vi "oef11.vi"() -> ()   [LabVIEW 2021]
uses:
  <vilib>/httpClient/LabVIEWHTTPClient.lvlib
panel:
  out "before substring":string
  out "match substring":string
  out "after substring":string
  in  "word":string
  out "headers":string
  out "body":string
  in  "String":string
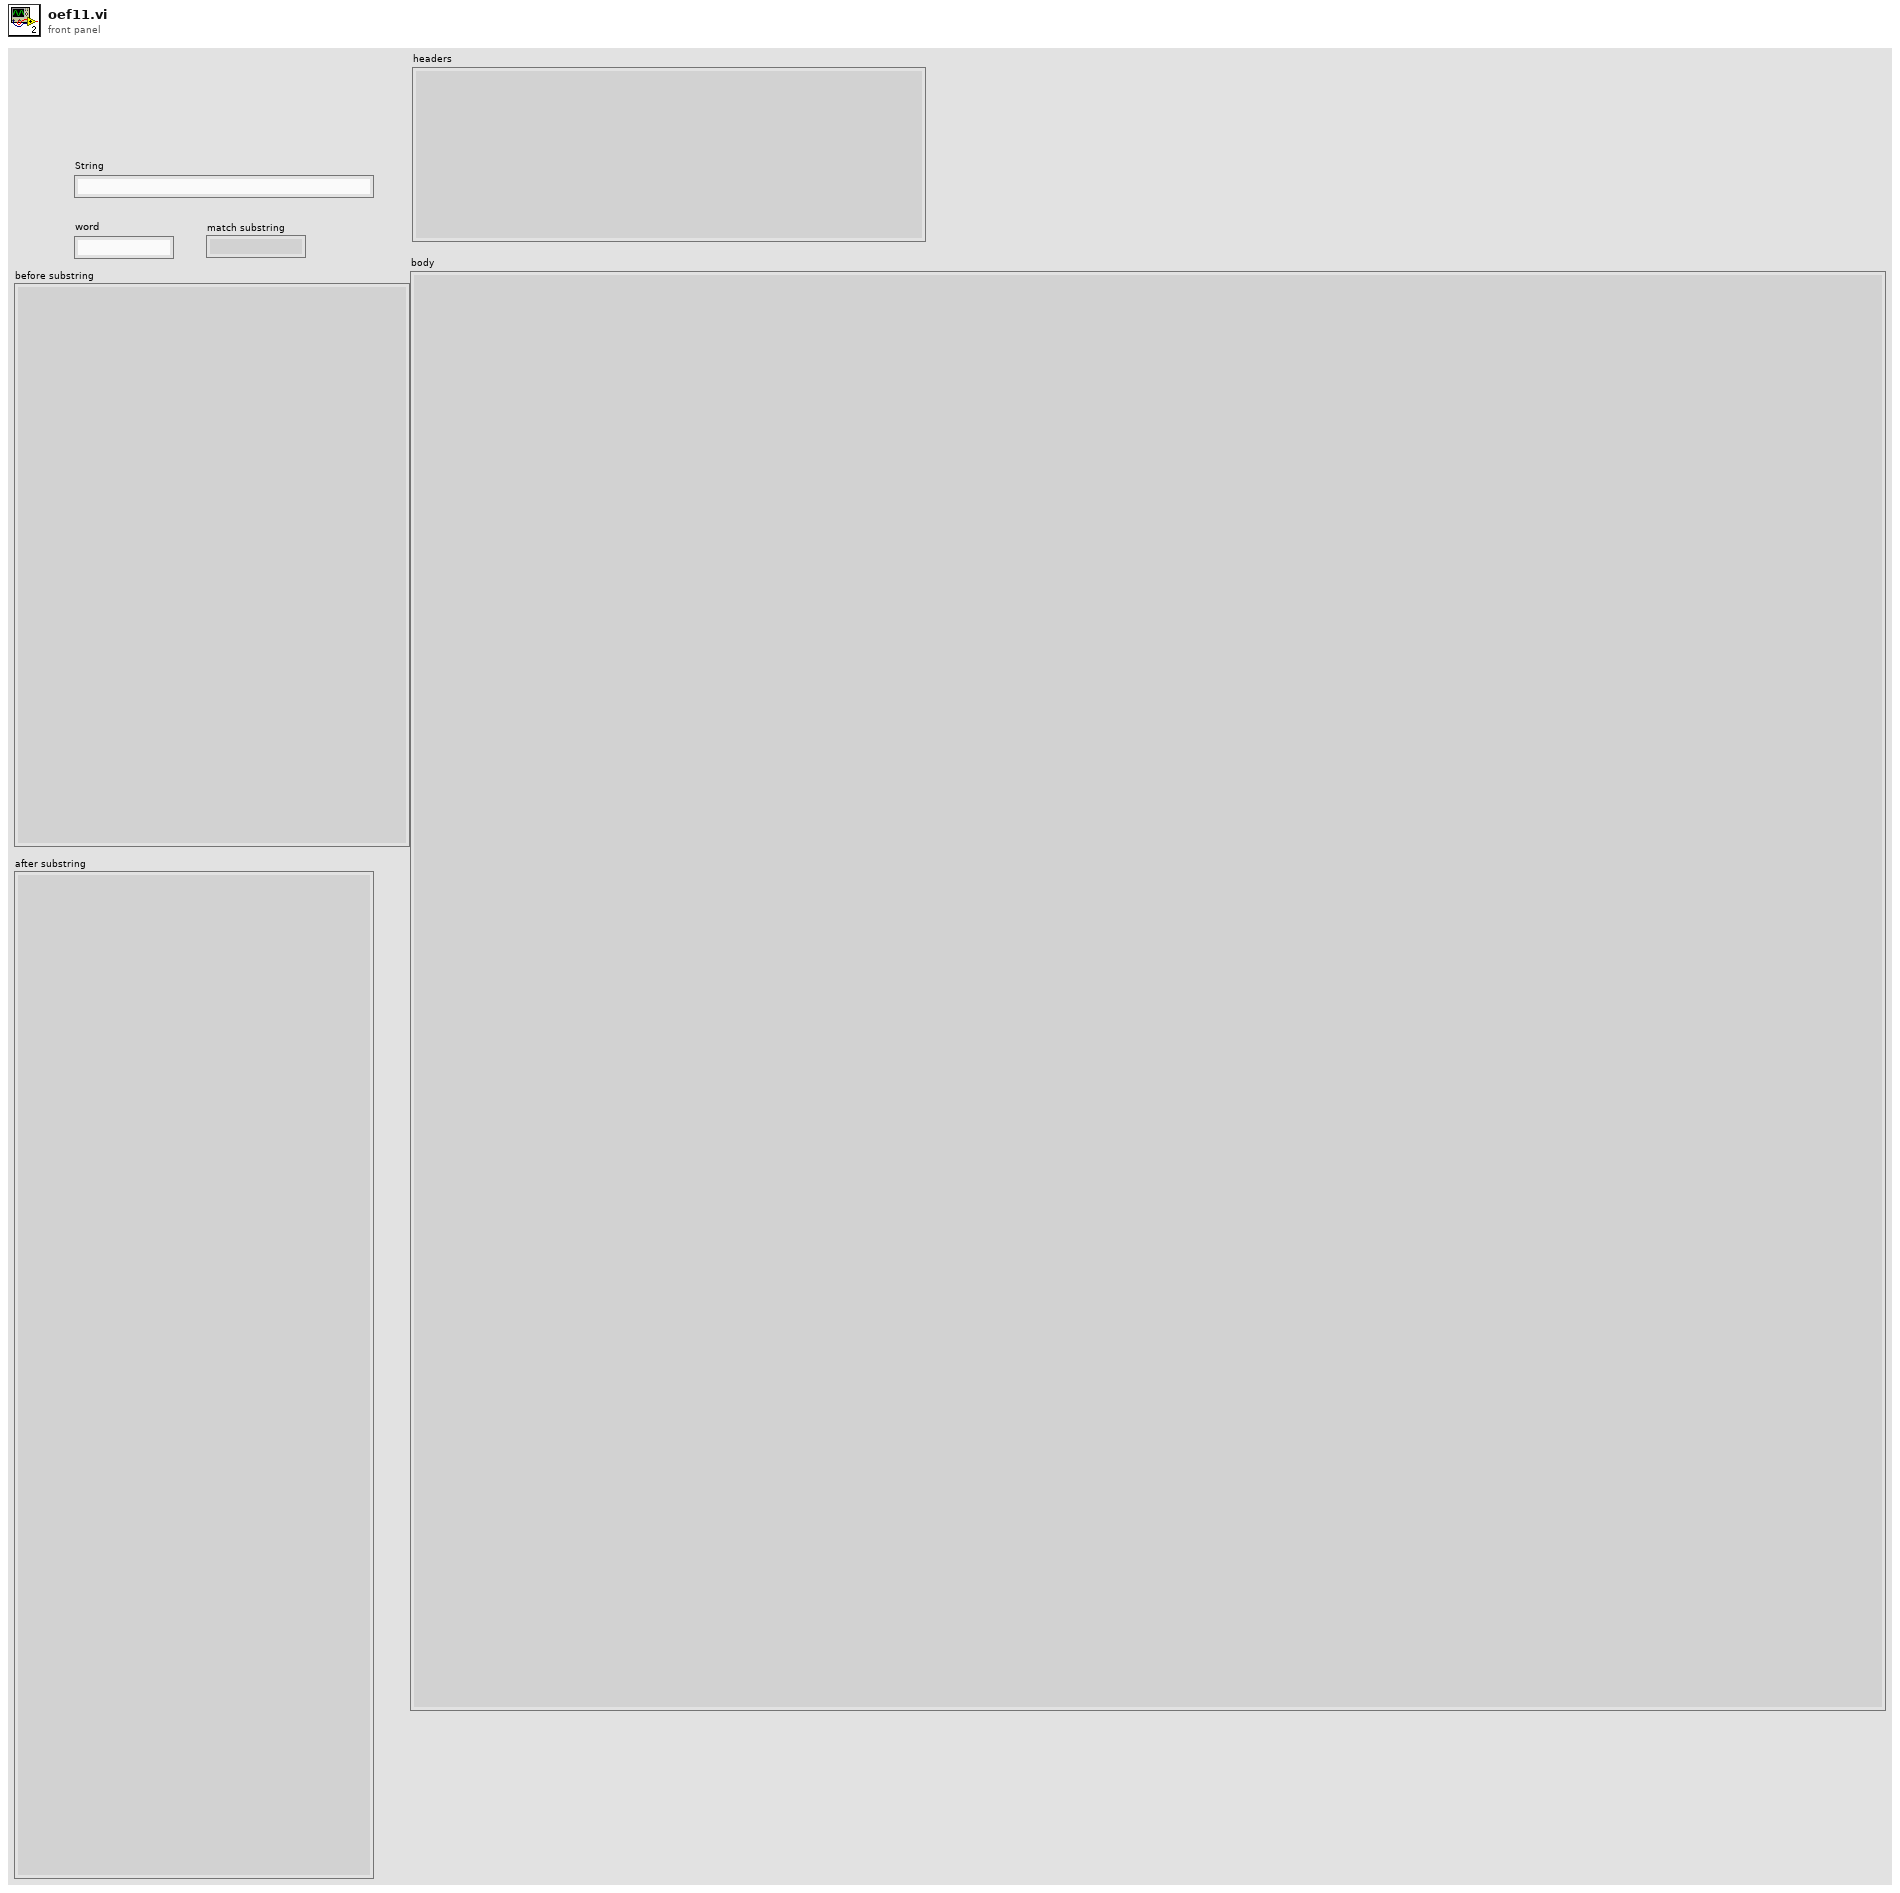
[diagram p1: front panel]
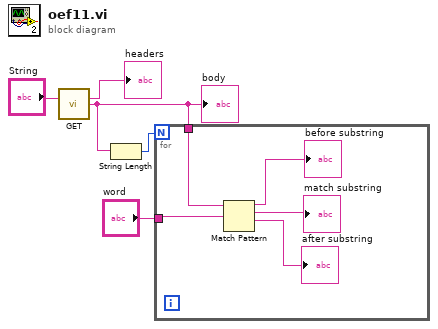
[diagram p0: block diagram]
diagram:
  n1 = call <vilib>:"GET.vi"("url"="String") -> ("headers"=→"headers":string, "body"=w2:string)  [unwired: 11 in, 2 out]
  "body" <- w2
  n2 = String Length(string=w2) -> (length=w3:i32)
  n3 = for {
    N: w3 -> [_]
    tunnel: w2 -> [w9]
    tunnel: "word" -> [w10]
    n4 = Match Pattern(string=w9, regular expression=w10) -> (before substring=→"before substring":string, match substring=→"match substring":string, after substring=→"after substring":string)  [unwired: 1 in, 1 out]
  }
